vi "CubicHermiteSpline_getControlVectorFromArrays.vi"(9 "finalVector":dbl[](array[numeric]), 11 "initialVector":dbl[](array[numeric])) -> (0 "error out":errorcluster, 3 "ControlVector":T1)   [LabVIEW 2019, in "Trajectory_Library.lvlib"]
doc: "Returns the control vector for each dimension as a matrix from the user-provided arrays in the constructor.\n\nParameters:\n - initialVector - The control vector for the initial point.\n - finalVector - The control vector for the final point.\n\nReturns:\n - ControlVector - The control vector matrix for a dimension.\n - Error Out - The output error cluster"
uses:
  Trajectory_Library.lvlib
  <vilib>/Analysis/Matrix/Datatypes/RealMatrix.ctl
  <vilib>/Analysis/Matrix/NI_Matrix.lvlib
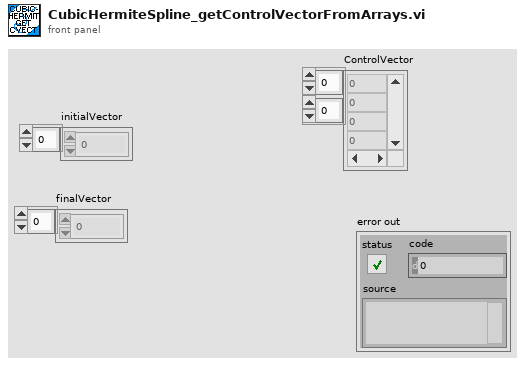
[diagram p1: front panel]
types:
  T1 = typedef "NI_Matrix.lvlib/RealMatrix.ctl" = dbl[][]
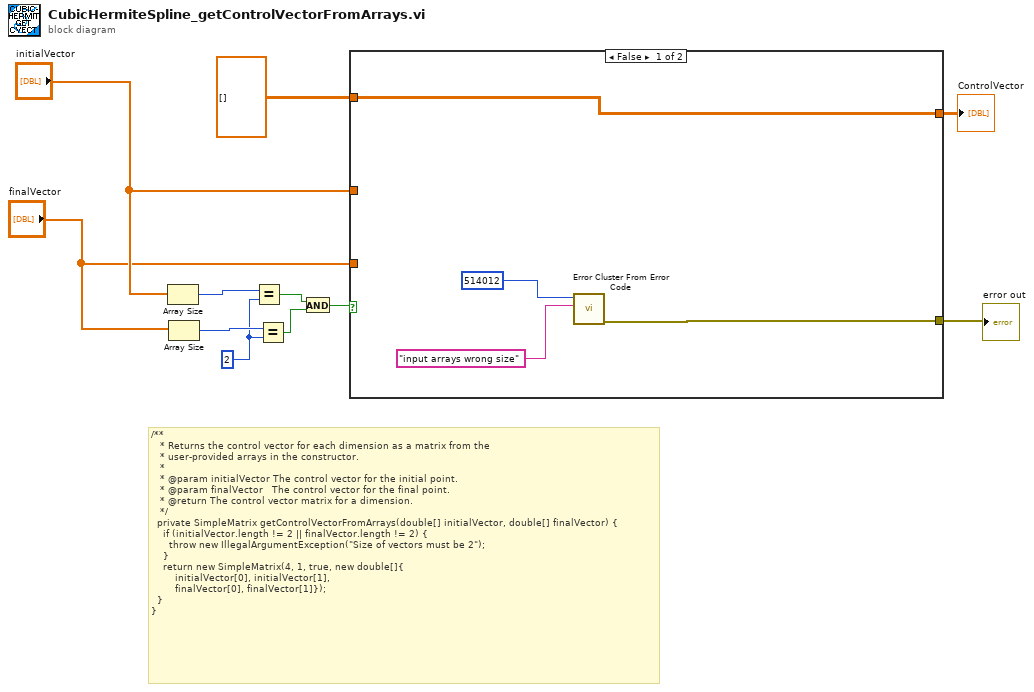
[diagram p0: block diagram]
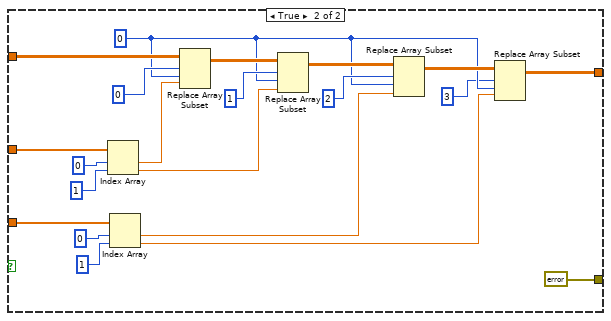
[diagram p2: hidden frame]
diagram:
  w9 = 2 ("y")
  # "/**\n   * Returns the control vector for each dimension as a matrix from the\n   * user-provided arrays in the constructor.\n   *\n   * @param initialVector The control vector for the initial point.\n   * @param finalVector   The control vector for the final point.\n   * @return The control vector matrix for a dimension.\n   */\n  private SimpleMatrix getControlVectorFromArrays(double[] initialVector, double[] finalVector) {\n    if (initialVector.length != 2 || finalVector.length != 2) {\n      throw new IllegalArgumentException(\"Size of vectors must be 2\");\n    }\n    return new SimpleMatrix(4, 1, true, new double[]{\n        initialVector[0], initialVector[1],\n        finalVector[0], finalVector[1]});\n  }\n}"
  n1 = Array Size(array="initialVector") -> (size(s)=w11:i32)
  n2 = Array Size(array="finalVector") -> (size(s)=w10:i32)
  n3 = Equal?(x=w11, y=w9) -> (x = y?=w8:bool)
  n4 = Equal?(x=w10, y=w9) -> (x = y?=w7:bool)
  n5 = And(x=w8, y=w7) -> (x .and. y?=w6:bool)
  n6 = case shown="False" w6 {
    tunnel: [w15 errorcluster {"status"=FALSE, "code"=0, "source"=""} ("error out")] -> w5
    tunnel: [w12 w30] -> w4
    tunnel: T1 [] ("ControlVector") -> [w12 w35]
    tunnel: "initialVector" -> [_ w25]
    tunnel: "finalVector" -> [_ w22]
    frame False {
      n7 = call <vilib>:"Error Cluster From Error Code.vi"("error message (\"\")"="input arrays wrong size" ("error message (\"\")"), "error code (0)"=514012) -> ("error out"=w15:errorcluster)  [unwired: 7 in]
    }
    frame True {
      w27 = 0 ("disabled index (col)")
      n8 = Index Array(array=w25, index #1=0 ("index"), index #2=1 ("index")) -> (element #1=w21:dbl, element #2=w20:dbl)
      n9 = Index Array(array=w22, index #1=0 ("index"), index #2=1 ("index")) -> (element #1=w19:dbl, element #2=w18:dbl)
      n10 = Replace Array Subset(array=w35, new element=w21, index (row)=0 ("disabled index (row)"), index (col)=w27) -> (w33:T1)
      n11 = Replace Array Subset(array=w33, new element=w20, index (row)=1 ("disabled index (row)"), index (col)=w27) -> (w32:T1)
      n12 = Replace Array Subset(array=w32, new element=w19, index (row)=2 ("disabled index (row)"), index (col)=w27) -> (w31:T1)
      n13 = Replace Array Subset(array=w31, new element=w18, index (row)=3 ("disabled index (row)"), index (col)=w27) -> (w30:T1)
    }
  }
  "ControlVector" <- w4
  "error out" <- w5
